vi "Create or Add Phrase or Paragraph.vi"(0 "Phrase refnum IN":refnum<k24>, 2 "Phrase or paragraph":T1, 5 "Paragraph refnum IN":refnum<k24>, 7 "Font refnum":refnum<k24>, 9 "value":refnum<k24>, 11 "error in (no error)":errorcluster, 12 "Leading":sgl=12.0, 13 "Only":enum16{"Create", "Append"}(ring)) -> (4 "Phrase refnum OUT":refnum<k24>, 6 "Paragraph refnum OUT":refnum<k24>, 15 "error out":errorcluster)   [LabVIEW 2019, in "Exaprom PDF.lvlib"]
doc: "Version 2.0\nDeveloped by Jean-Marc Simard\nCopyright © 2012, Exaprom Inc.\nAll rights reserved.\nLicense: BSD\n\nWith iTextSharp 4.1.6 (http://itextsharp.sourceforge.net)\nunder Mozilla Public License Version 1.1\n(http://www.mozilla.org/MPL/MPL-1.1.html)"
uses:
  Controls/Text Controls/Phrase or paragraph.ctl
  C:/work/niobrara_lv/labview pdf writer fixing/DLL/itextsharp.dll
  DLL/itextsharp.dll
  Exaprom PDF.lvlib
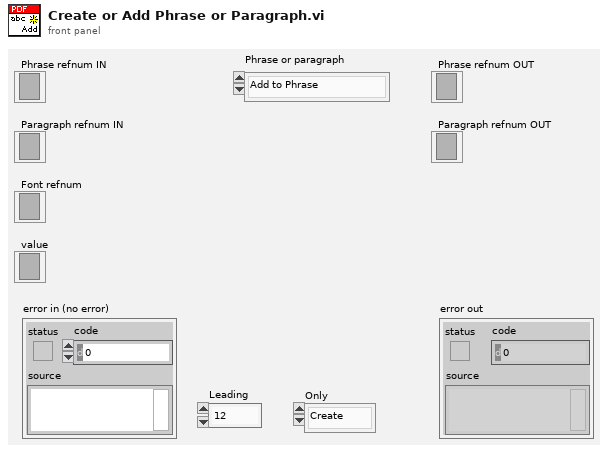
[diagram p1: front panel]
types:
  T1 = typedef "Exaprom PDF.lvlib/Phrase or paragraph.ctl" = enum16{"Add to Phrase", "Add to Paragraph", "Create Phrase", "Create Paragraph"}
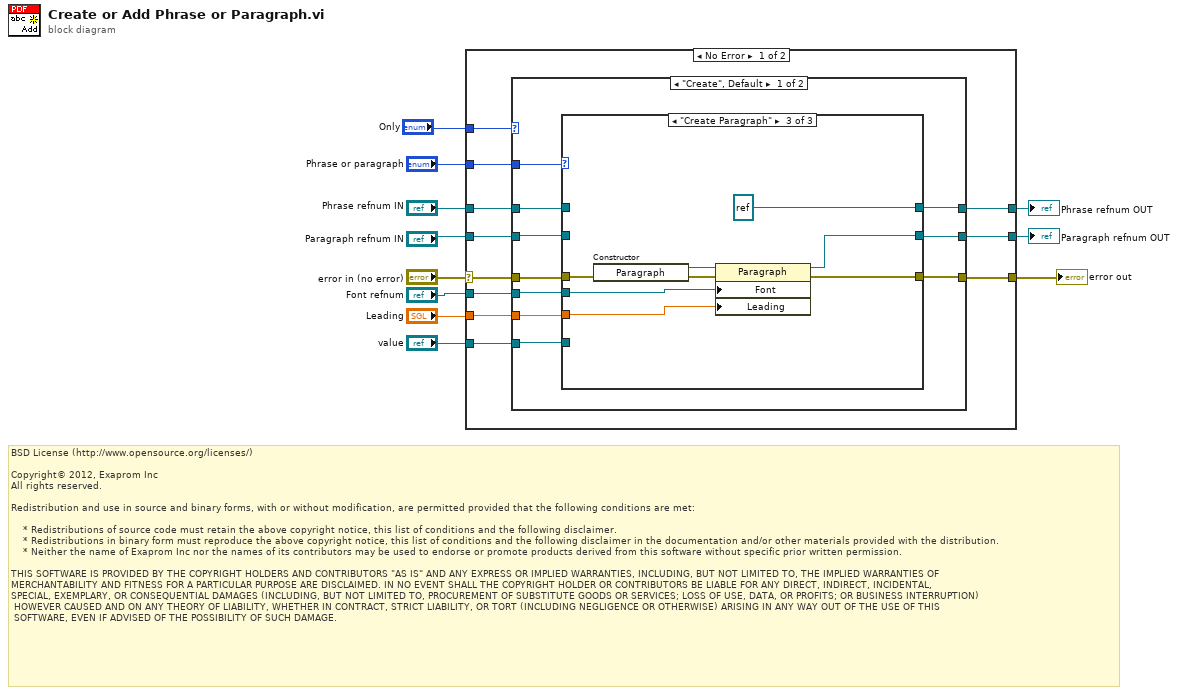
[diagram p0: block diagram]
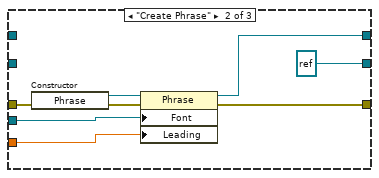
[diagram p3: hidden frame]
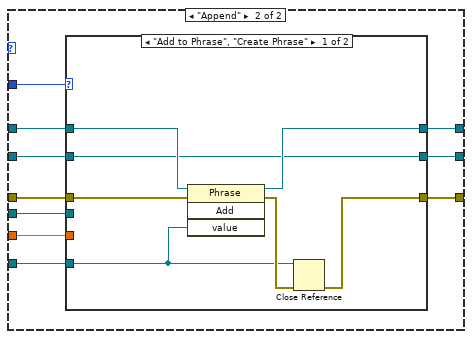
[diagram p4: hidden frame]
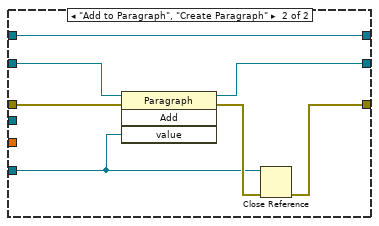
[diagram p5: hidden frame]
diagram:
  # "BSD License (http://www.opensource.org/licenses/)\n\nCopyright© 2012, Exaprom Inc\nAll rights reserved.\n\nRedistribution and use in source and binary forms, with or without modification, are permitted provided that the following conditions are met:\n\n    * Redistributions of source code must retain the above copyright notice, this list of conditions and the following disclaimer.\n    * Redistributions in binary form must reproduce the above copyright notice, this list of conditions and the following disclaimer in the documentation and/or other materials provided with the distribution.\n    * Neither the name of Exaprom Inc nor the names of its contributors may be used to endorse or promote products derived from this software without specific prior written permission.\n\nTHIS SOFTWARE IS PROVIDED BY THE COPYRIGHT HOLDERS AND CONTRIBUTORS \"AS IS\" AND ANY EXPRESS OR IMPLIED WARRANTIES, INCLUDING, BUT NOT LIMITED TO, THE IMPLIED WARRANTIES OF \nMERCHANTABILITY AND FITNESS FOR A PARTICULAR PURPOSE ARE DISCLAIMED. IN NO EVENT SHALL THE COPYRIGHT HOLDER OR CONTRIBUTORS BE LIABLE FOR ANY DIRECT, INDIRECT, INCIDENTAL,\nSPECIAL, EXEMPLARY, OR CONSEQUENTIAL DAMAGES (INCLUDING, BUT NOT LIMITED TO, PROCUREMENT OF SUBSTITUTE GOODS OR SERVICES; LOSS OF USE, DATA, OR PROFITS; OR BUSINESS INTERRUPTION)\n HOWEVER CAUSED AND ON ANY THEORY OF LIABILITY, WHETHER IN CONTRACT, STRICT LIABILITY, OR TORT (INCLUDING NEGLIGENCE OR OTHERWISE) ARISING IN ANY WAY OUT OF THE USE OF THIS\n SOFTWARE, EVEN IF ADVISED OF THE POSSIBILITY OF SUCH DAMAGE."
  n1 = case shown="No Error" "error in (no error)" {
    selector: "error in (no error)" -> [w17 w78]
    tunnel: [w15 w78] -> w11
    tunnel: "Leading" -> [w22 _]
    tunnel: "Phrase refnum IN" -> [w21 w77]
    tunnel: "Paragraph refnum IN" -> [w20 w76]
    tunnel: "Phrase or paragraph" -> [w19 _]
    tunnel: "value" -> [w18 _]
    tunnel: "Font refnum" -> [w16 _]
    tunnel: [w14 w77] -> w3
    tunnel: [w13 w76] -> w2
    tunnel: "Only" -> [w12 _]
    frame No Error {
      n2 = case shown="\"Create\", Default" w12 {
        tunnel: w22 -> [w24 w61]
        tunnel: w21 -> [w30 w60]
        tunnel: w20 -> [w31 w59]
        tunnel: w19 -> [w29 w58]
        tunnel: w18 -> [w25 w57]
        tunnel: w17 -> [w32 w56]
        tunnel: w16 -> [w23 w55]
        tunnel: [w26 w54] -> w15
        tunnel: [w28 w53] -> w14
        tunnel: [w27 w52] -> w13
        frame "Create", Default {
          n3 = case shown="\"Create Paragraph\"" w29 {
            tunnel: [w33 w41 w49] -> w26
            tunnel: [w34 refnum<k24> refnum ("new reference") w47] -> w27
            tunnel: w24 -> [_ w40 w48]
            tunnel: w30 -> [w35 _ _]
            tunnel: w31 -> [w34 _ _]
            tunnel: w32 -> [w33 w39 w45]
            tunnel: w25 -> [_ _ _]
            tunnel: [w35 w38 refnum<k24> refnum ("new reference")] -> w28
            tunnel: w23 -> [_ w37 w46]
            frame "Add to Phrase", "Add to Paragraph" {
            }
            frame "Create Phrase" {
              n4 = constructor class="Phrase"(error in=w39) -> (reference out=w43:refnum<k24>, error out=w42:errorcluster)  [unwired: 2 in, 1 out]
              n5 = property class="Phrase"(reference=w43, error in=w42, "Font"=w37, "Leading"=w40) -> (reference out=w38:refnum<k24>, error out=w41:errorcluster)
            }
            frame "Create Paragraph" {
              n6 = constructor class="Paragraph"(error in=w45) -> (reference out=w50:refnum<k24>, error out=w51:errorcluster)  [unwired: 2 in, 1 out]
              n7 = property class="Paragraph"(reference=w50, error in=w51, "Font"=w46, "Leading"=w48) -> (reference out=w47:refnum<k24>, error out=w49:errorcluster)
            }
          }
        }
        frame "Append" {
          n8 = case shown="\"Add to Phrase\", \"Create Phrase\"" w58 {
            tunnel: [w66 w73] -> w54
            tunnel: [w63 w69] -> w52
            tunnel: w61 -> [_ _]
            tunnel: w60 -> [w65 w71]
            tunnel: w59 -> [w63 w70]
            tunnel: w56 -> [w68 w75]
            tunnel: w57 -> [w62 w72]
            tunnel: [w64 w71] -> w53
            tunnel: w55 -> [_ _]
            frame "Add to Phrase", "Create Phrase" {
              n9 = invoke class="Phrase" method="Add"(reference=w65, error in=w68, "value"=w62) -> (reference out=w64:refnum<k24>, error out=w67:errorcluster)  [unwired: 1 in, 2 out]
              n10 = Close Reference(reference=w62, error in (no error)=w67) -> (error out=w66:errorcluster)
            }
            frame "Add to Paragraph", "Create Paragraph" {
              n11 = invoke class="Paragraph" method="Add"(reference=w70, error in=w75, "value"=w72) -> (reference out=w69:refnum<k24>, error out=w74:errorcluster)  [unwired: 1 in, 2 out]
              n12 = Close Reference(reference=w72, error in (no error)=w74) -> (error out=w73:errorcluster)
            }
          }
        }
      }
    }
    frame Error {
    }
  }
  "error out" <- w11
  "Phrase refnum OUT" <- w3
  "Paragraph refnum OUT" <- w2
